vi "Log to error file.vi"(8 "error in (no error)":errorcluster, 11 "Error info":T1) -> (0 "error out":errorcluster)   [LabVIEW 2017, in "Error.lvlib"]
uses:
  Error.lvlib
  ctl/ErrorInfo.ctl
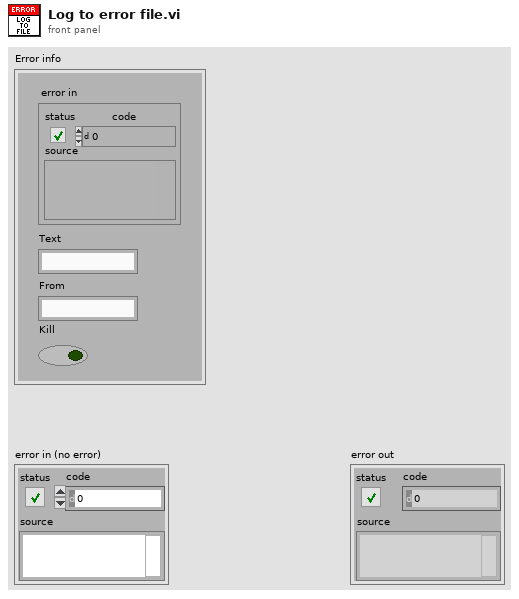
[diagram p1: front panel]
types:
  T1 = typedef "Error.lvlib/ErrorInfo.ctl" = cluster{"error in":errorcluster, "Text":string, "From":string, "Kill":bool}
  T2 = enum16{"open", "replace", "create", "open or create", "replace or create", "replace or create with confirmation"}
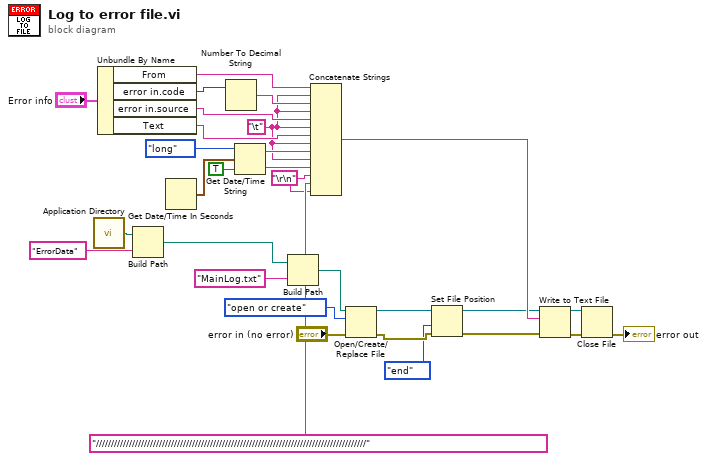
[diagram p0: block diagram]
diagram:
  w1 = "\r\n"
  w10 = "\t"
  n1 = call <vilib>:"Application Directory.vi"() -> ("Application Directory"=w30:path)
  n2 = Unbundle By Name("Error info") -> ("From"=w19:string, "error in.code"=w18:i32, "error in.source"=w16:string, "Text"=w15:string)
  n3 = Build Path(base path=w30, name or relative path="ErrorData") -> (appended path=w27:path)
  n4 = Get Date/Time In Seconds() -> (seconds since 1Jan1904=w14:timestamp)
  n5 = Number To Decimal String(number=w18) -> (decimal integer string=w17:string)  [unwired: 1 in]
  n6 = Get Date/Time String(date format (0)=enum16{"short", "long", "abbreviated"}."long", seconds (now)=w14, want seconds? (F)=TRUE) -> (date string=w11:string, time string=w9:string)
  n7 = Build Path(base path=w27, name or relative path="MainLog.txt") -> (appended path=w26:path)
  n8 = Concatenate Strings(w19, w10, w17, w10, w16, w10, w15, w10, w11, w10, w9, w1, "//////////////////////////////////////////////////////////////////////////////////////////" ("string"), w1) -> (w8:string)
  n9 = Open/Create/Replace File(file path (use dialog)=w26, error in="error in (no error)", operation (0:open)=T2."open or create") -> (refnum out=w6:refnum<file>, error out=w7:errorcluster)  [unwired: 3 in, 1 out]
  n10 = Set File Position(refnum=w6, from (0:start)=enum16{"start", "end", "current"}."end", error in=w7) -> (refnum out=w3:refnum<file>, error out=w4:errorcluster)  [unwired: 1 in]
  n11 = Write to Text File(file (use dialog)=w3, text=w8, error in=w4) -> (refnum out=w22:refnum<file>, error out=w23:errorcluster)  [unwired: 1 in, 1 out]
  n12 = Close File(refnum=w22, error in=w23) -> (error out=→"error out":errorcluster)  [unwired: 1 out]
